vi "getTodayFolderRemote.vi"(8 "error in (no error)":errorcluster, 11 "FileNeologist in":refnum<class "FileNeologist.lvclass">) -> (0 "error out":errorcluster, 2 "todayFolder":path, 3 "FileNeologist out":refnum<class "FileNeologist.lvclass">)   [LabVIEW 2009, in "Tools.lvlib" / "Filing.lvlib" / "FileNeologist.lvclass"]
uses:
  FileNeologist.lvclass
  FileNeologist.lvclass/FileNeologist.ctl
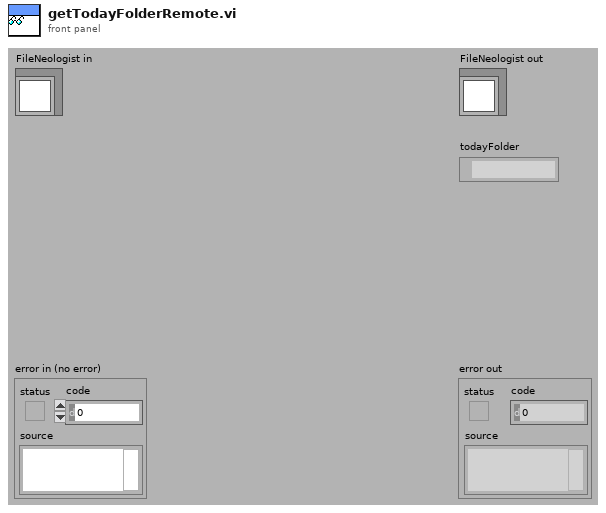
[diagram p1: front panel]
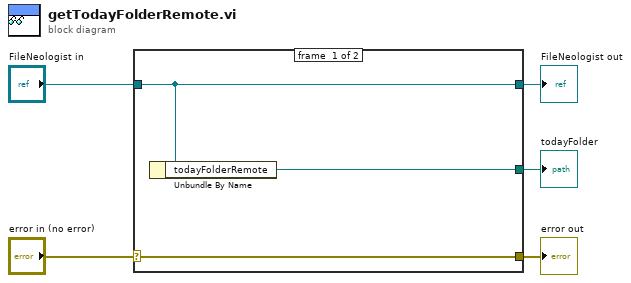
[diagram p0: block diagram]
diagram:
  n1 = case shown="No Error" "error in (no error)" {
    selector: "error in (no error)" -> [w8 w9]
    tunnel: [w8 w9] -> w4
    tunnel: [w7 w10] -> w2
    tunnel: "FileNeologist in" -> [w7 w10]
    tunnel: [w6 _] -> w1
    frame #0 {
      n2 = Unbundle By Name(w7) -> ("todayFolderRemote"=w6:path)
    }
    frame #1 {
    }
  }
  "error out" <- w4
  "FileNeologist out" <- w2
  "todayFolder" <- w1
